vi "Move Sequence.vi"(8 "Distance Up":dbl=28.0, 11 "Distance Down":dbl=28.0) -> ()   [LabVIEW 2014]
uses:
  Begin/Global Variables.vi
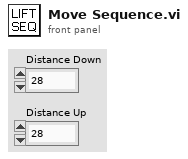
[diagram p1: front panel]
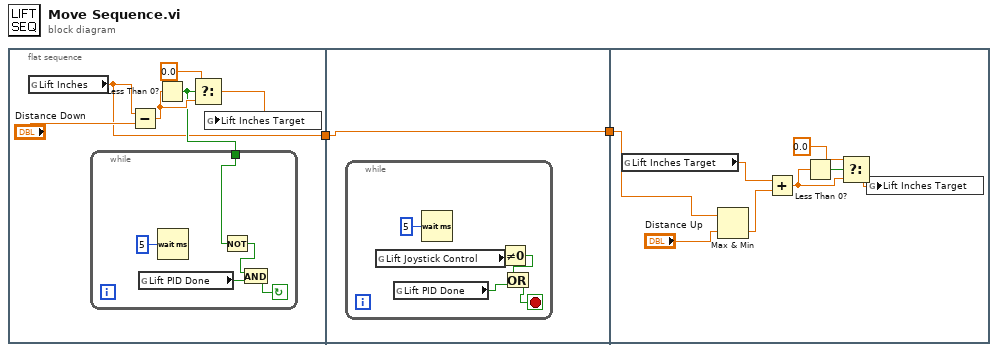
[diagram p0: block diagram]
diagram:
  n1 = flat-sequence {
    tunnel: [w3] -> w1
    tunnel: [w14] -> w2
    tunnel: w1 -> [w14]
    tunnel: w2 -> [w20]
    frame #0 {
      n2 = global read "Global Variables.vi" "Lift Inches"() -> (w3:dbl)
      n3 = Subtract(x=w3, y="Distance Down") -> (x-y=w7:dbl)
      n4 = Less Than 0?(x=w7) -> (x < 0?=w4:bool)
      n5 = while {
        tunnel: w4 -> [w9]
        stop <- w11 continue-if-true
        n6 = global read "Global Variables.vi" "Lift PID Done"() -> (w12:bool)
        n7 = Wait (ms)(milliseconds to wait=u32 5) -> ()  [unwired: 1 out]
        n8 = Not(x=w9) -> (.not. x?=w10:bool)
        n9 = And(x=w10, y=w12) -> (x .and. y?=w11:bool)
      }
      n10 = Select(t=0.0, s=w4, f=w7) -> (s? t:f=w6:dbl)
      n11 = global write "Global Variables.vi" "Lift Inches Target"(w6) -> ()
    }
    frame #1 {
      n12 = while {
        stop <- w15 stop-if-true
        n13 = global read "Global Variables.vi" "Lift Joystick Control"() -> (w17:dbl)
        n14 = global read "Global Variables.vi" "Lift PID Done"() -> (w18:bool)
        n15 = Wait (ms)(milliseconds to wait=u32 5) -> ()  [unwired: 1 out]
        n16 = Not Equal To 0?(x=w17) -> (x != 0?=w16:bool)
        n17 = Or(x=w16, y=w18) -> (x .or. y?=w15:bool)
      }
    }
    frame #2 {
      n18 = global read "Global Variables.vi" "Lift Inches Target"() -> (w25:dbl)
      n19 = Max & Min(x=w20, y="Distance Up") -> (min(x,y)=w21:dbl)  [unwired: 1 out]
      n20 = Add(x=w25, y=w21) -> (x+y=w26:dbl)
      n21 = Less Than 0?(x=w26) -> (x < 0?=w27:bool)
      n22 = Select(t=0.0, s=w27, f=w26) -> (s? t:f=w24:dbl)
      n23 = global write "Global Variables.vi" "Lift Inches Target"(w24) -> ()
    }
  }
